vi "oa_Generate Cursor List for SCL Plot.vi"(6 "label settings":T4={"show label? (Y)"=TRUE, "avoid overlap? (Y)"=TRUE}, 7 "cursor attributes":T3={"layout color"=852223, "active color"=16740820, "precision"=2, "BG transparent? (T)"=TRUE, "radius"=2}, 8 "error in (no error)":errorcluster, 9 "Max number of labels\nalong radius":i32=5, 10 "scale":T1, 11 "DC Gap":cluster{"X":dbl[], "Y":dbl[]}[](array[cluster]) {"Y" format="%.2f"; "X" format="%.2f"}) -> (0 "error out":errorcluster, 2 "Cursor List (EU position]":T2(array[cluster]) {"Location"."phase" format="%.2f"; "Location"."mag" format="%.2f"}, 3 "DC Gap out":cluster{"X":dbl[], "Y":dbl[]}[](array[cluster]) {"Y" format="%.2f"; "X" format="%.2f"})   [LabVIEW 2017]
uses:
  <vilib>/addons/Sound and Vibration/Order Analysis/Backward Compatibility/SubVIs/OAT Polar Cursor Attributes.ctl
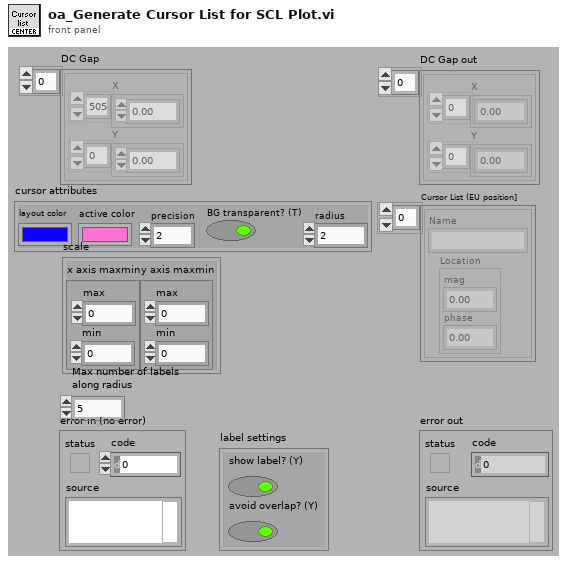
[diagram p1: front panel]
types:
  T1 = cluster{"x axis maxmin":cluster{"max":dbl, "min":dbl}, "y axis maxmin":cluster{"max":dbl, "min":dbl}}
  T2 = cluster{"Name":string, "Location":cluster{"mag":dbl, "phase":dbl}}[]
  T3 = typedef "OAT Polar Cursor Attributes.ctl" = cluster{"layout color":u32, "active color":u32, "precision":i16, "BG transparent? (T)":bool, "radius":i16}
  T4 = cluster{"show label? (Y)":bool, "avoid overlap? (Y)":bool}
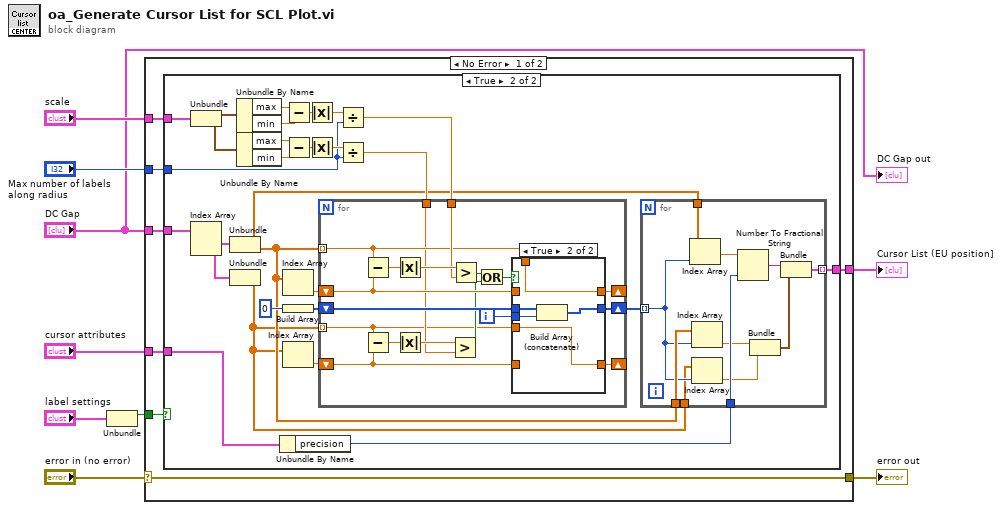
[diagram p0: block diagram]
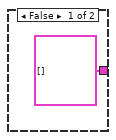
[diagram p2: hidden frame]
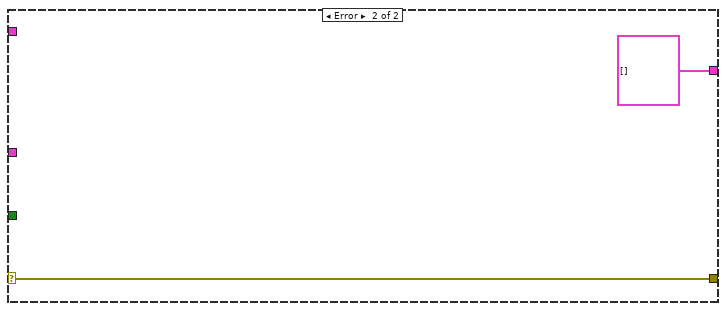
[diagram p4: hidden frame]
diagram:
  n1 = Unbundle("label settings") -> ("show label? (Y)"=w5:bool)  [unwired: 1 out]
  n2 = case shown="No Error" "error in (no error)" {
    selector: "error in (no error)" -> [w16 w84]
    tunnel: [w16 w84] -> w8
    tunnel: "Max number of labels\nalong radius" -> [w15 _]
    tunnel: w5 -> [w14 _]
    tunnel: "scale" -> [w13 _]
    tunnel: "DC Gap" -> [w12 _]
    tunnel: [w11 cluster{string, cluster{dbl, dbl}}[] []] -> w3
    tunnel: "cursor attributes" -> [w10 _]
    frame No Error {
      n3 = case shown="True" w14 {
        tunnel: w15 -> [_ w28]
        tunnel: w13 -> [_ w36]
        tunnel: w12 -> [_ w26]
        tunnel: [cluster{string, cluster{dbl, dbl}}[] [] w21] -> w11
        tunnel: w10 -> [_ w18]
        frame False {
        }
        frame True {
          n4 = Unbundle(w36) -> ("x axis maxmin"=w35:cluster{"max":dbl, "min":dbl}, "y axis maxmin"=w34:cluster{"max":dbl, "min":dbl})
          n5 = Index Array(array=w26) -> (element #1=w25:cluster{"X":dbl[], "Y":dbl[]}, element #2=w24:cluster{"X":dbl[], "Y":dbl[]})  [unwired: 2 in]
          n6 = Unbundle(w25) -> ("X"=w23:dbl[], "Y"=w22:dbl[])
          n7 = Unbundle(w24) -> ("Y"=w19:dbl[])  [unwired: 1 out]
          n8 = Unbundle By Name(w35) -> ("max"=w45:dbl, "min"=w44:dbl)
          n9 = Unbundle By Name(w34) -> ("max"=w30:dbl, "min"=w29:dbl)
          n10 = Unbundle By Name(w18) -> ("precision"=w42:i16)
          n11 = Index Array(array=w22) -> (element=w38:dbl)  [unwired: 1 in]
          n12 = Build Array(0 ("element")) -> (w40:i32[])
          n13 = Index Array(array=w19) -> (element=w20:dbl)  [unwired: 1 in]
          n14 = Subtract(x=w45, y=w44) -> (x-y=w31:dbl)
          n15 = Subtract(x=w30, y=w29) -> (x-y=w32:dbl)
          n16 = Absolute Value(x=w31) -> (abs(x)=w43:dbl)
          n17 = Absolute Value(x=w32) -> (abs(x)=w33:dbl)
          n18 = Divide(x=w43, y=w28) -> (x/y=w39:dbl)
          n19 = Divide(x=w33, y=w28) -> (x/y=w27:dbl)
          n20 = for {
            tunnel: w39 -> [w61]
            shift-right: [w59] -> w41
            shift-left: w40 -> [w60]
            tunnel: w22 -> [w58] mode=indexing
            shift-right: [w57] -> _
            shift-left: w38 -> [w56]
            tunnel: w27 -> [w50]
            shift-right: [w53] -> _
            shift-left: w20 -> [w54]
            tunnel: w19 -> [w46] mode=indexing
            i -> [w55]
            n21 = Subtract(x=w58, y=w56) -> (x-y=w63:dbl)
            n22 = Subtract(x=w46, y=w54) -> (x-y=w52:dbl)
            n23 = Absolute Value(x=w63) -> (abs(x)=w62:dbl)
            n24 = Absolute Value(x=w52) -> (abs(x)=w51:dbl)
            n25 = Greater?(x=w51, y=w50) -> (0:w48:bool)
            n26 = Greater?(x=w62, y=w61) -> (0:w49:bool)
            n27 = Or(x=w49, y=w48) -> (x .or. y?=w47:bool)
            n28 = case shown="True" w47 {
              tunnel: w60 -> [w66 w71]
              tunnel: w58 -> [_ w68]
              tunnel: [w66 w70] -> w59
              tunnel: [w65 w68] -> w57
              tunnel: w56 -> [w65 _]
              tunnel: w55 -> [_ w69]
              tunnel: w54 -> [w64 _]
              tunnel: [w64 w67] -> w53
              tunnel: w46 -> [_ w67]
              frame False {
              }
              frame True {
                n29 = Build Array (concatenate)(w71, w69) -> (w70:i32[])
              }
            }
          }
          n30 = for {
            tunnel: w42 -> [w82]
            tunnel: w41 -> [w75] mode=indexing
            tunnel: [w79] -> w21 mode=indexing
            tunnel: w23 -> [w77]
            tunnel: w22 -> [w76]
            tunnel: w19 -> [w74]
            n31 = Index Array(array=w77, index=w75) -> (element=w78:dbl)
            n32 = Index Array(array=w76, index=w75) -> (element=w73:dbl)
            n33 = Index Array(array=w74, index=w75) -> (element=w72:dbl)
            n34 = Number To Fractional String(number=w78, precision (6)=w82) -> (F-format string=w81:string)  [unwired: 2 in]
            n35 = Bundle(w73, w72) -> (w80:cluster{dbl, dbl})  [unwired: 1 in]
            n36 = Bundle(w81, w80) -> (w79:cluster{string, cluster{dbl, dbl}})  [unwired: 1 in]
          }
        }
      }
    }
    frame Error {
    }
  }
  "error out" <- w8
  "Cursor List (EU position]" <- w3
  "DC Gap out" <- "DC Gap"
